vi "Verify Response.vi"(7 "Timeout (ms)":dbl, 8 "error in (no error)":errorcluster, 10 "output cluster in":T1, 11 "VISA Refnum in":refnum<visa-resource-name>) -> (0 "error out":errorcluster, 2 "output cluster out":T1, 3 "VISA Refnum out":refnum<visa-resource-name>)   [LabVIEW 2020]
uses:
  Data Cluster.ctl
panel:
  # "Send Data:"
  # "Receive Data:"
  # "Send Data:"
  # "Receive Data:"
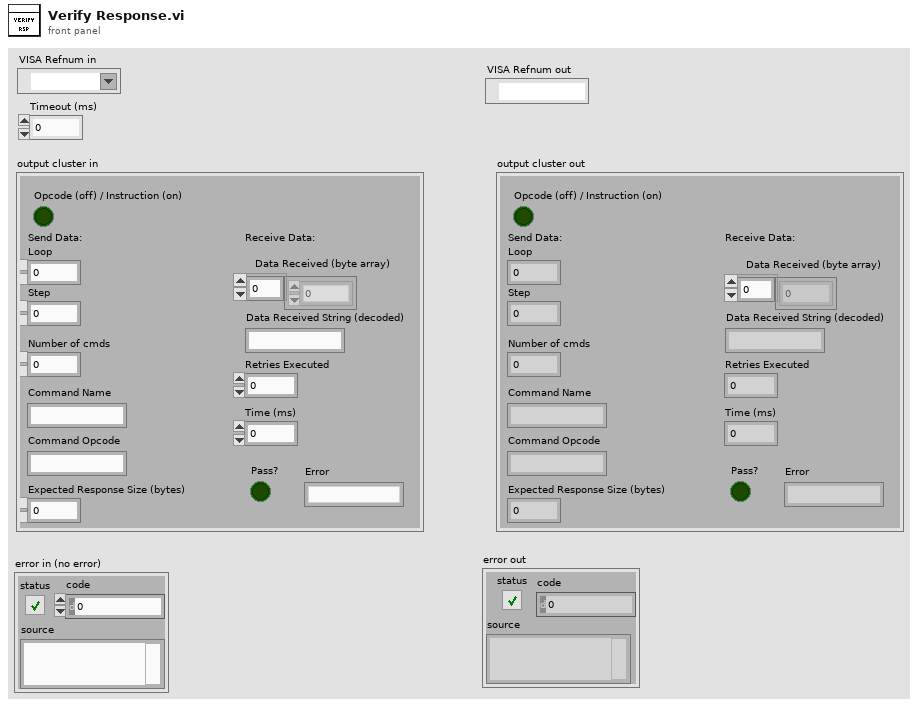
[diagram p1: front panel]
types:
  T1 = typedef "Data Cluster.ctl" = cluster{"Command Name":string, "Command Opcode ":string, "Step":dbl, "Loop":dbl, "Expected Response Size (bytes)":u16, "Number of cmds":dbl, "Data Received (byte array)":u8[], "Retries Executed":u16, "Time (ms)":u16, "Pass?":bool, "Opcode (off) / Instruction (on)":bool, "Data Received String (decoded)":string, "Error":string}
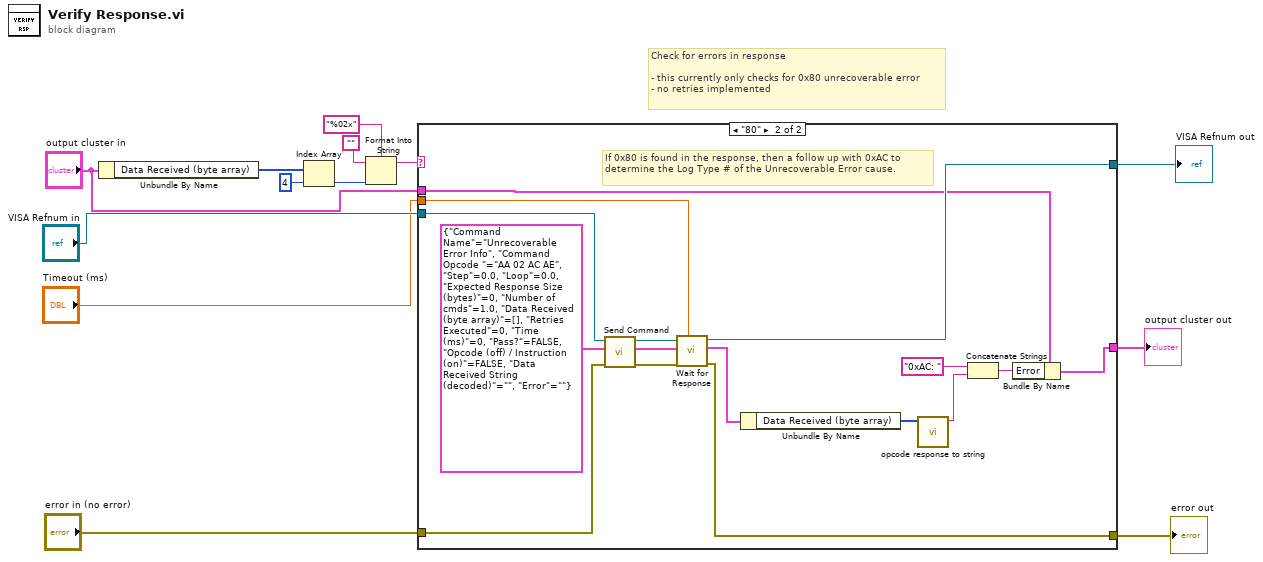
[diagram p0: block diagram]
diagram:
  # "Check for errors in response\n\n- this currently only checks for 0x80 unrecoverable error\n- no retries implemented"
  n1 = Unbundle By Name("output cluster in") -> ("Data Received (byte array)"=w12:u8[])
  n2 = Index Array(array=w12, index=4) -> (element=w9:u8)
  n3 = Format Into String(format string="%02x", initial string="", w9) -> (resulting string=w8:string)  [unwired: 1 in, 1 out]
  n4 = case shown="\"80\"" w8 {
    tunnel: "VISA Refnum in" -> [w14 w31]
    tunnel: "Timeout (ms)" -> [_ w29]
    tunnel: "error in (no error)" -> [w16 w27]
    tunnel: [w14 w25] -> w4
    tunnel: [w15 w18] -> w3
    tunnel: [w16 w24] -> w2
    tunnel: "output cluster in" -> [w15 w17]
    frame Default {
    }
    frame "80" {
      # "If 0x80 is found in the response, then a follow up with 0xAC to determine the Log Type # of the Unrecoverable Error cause."
      n5 = call "Send Command.vi"("error in (no error)"=w27, "Data cluster in"=T1 {"Command Name"="Unrecoverable Error Info", "Command Opcode "="AA 02 AC AE", "Step"=0.0, "Loop"=0.0, "Expected Response Size (bytes)"=0, "Number of cmds"=1.0, "Data Received (byte array)"=[], "Retries Executed"=0, "Time (ms)"=0, "Pass?"=FALSE, "Opcode (off) / Instruction (on)"=FALSE, "Data Received String (decoded)"="", "Error"=""}, "VISA Refnum in"=w31) -> ("error out"=w26:errorcluster, "Data cluster out"=w28:T1, "VISA Refnum out"=w30:refnum<visa-resource-name>)  [unwired: 6 in]
      n6 = call "Wait for Response.vi"("Timeout (ms)"=w29, "error in (no error)"=w26, "Data cluster in"=w28, "VISA Refnum in"=w30) -> ("error out"=w24:errorcluster, "output cluster"=w21:T1, "VISA Refnum out"=w25:refnum<visa-resource-name>)  [unwired: 4 in, 1 out]
      n7 = Unbundle By Name(w21) -> ("Data Received (byte array)"=w20:u8[])
      n8 = call "opcode response to string.vi"("Data Received"=w20) -> ("Response String"=w19:string)  [unwired: 10 in]
      n9 = Concatenate Strings("0xAC: " ("string"), w19) -> (w22:string)
      n10 = Bundle By Name(cluster=w17, "Error"=w22) -> (w18:T1)
    }
  }
  "output cluster out" <- w3
  "error out" <- w2
  "VISA Refnum out" <- w4
